vi "select_data_points.vi"(0 "Total HCl masses":dbl[](array[numeric]), 1 "EMFs":dbl[](array[numeric]), 2 "E0":dbl, 3 "k":dbl, 4 "Sample Mass":dbl) -> (5 "EMF Array (pH3-3.5)":dbl[](array[numeric]), 6 "m/m0 Array":dbl[](array[numeric]), 7 "First Point":dbl, 8 "Last Point":dbl)   [LabVIEW 2010]
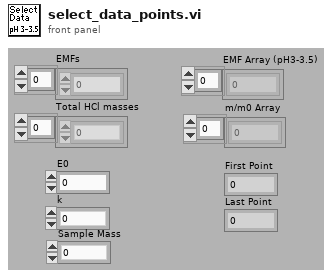
[diagram p1: front panel]
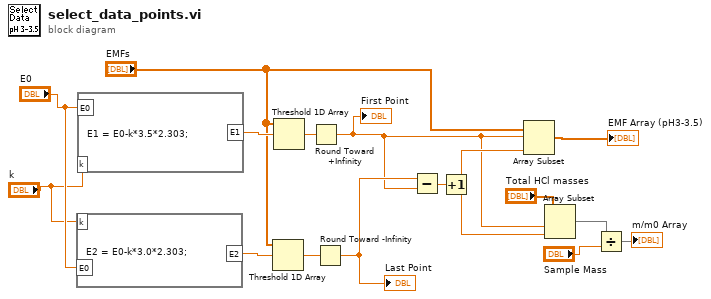
[diagram p0: block diagram]
diagram:
  n1 = formula code="E2 = E0-k*3.0*2.303;"("E0"="E0", "k"="k") -> ("E2"=w12:dbl)
  n2 = formula code="E1 = E0-k*3.5*2.303;"("E0"="E0", "k"="k") -> ("E1"=w13:dbl)
  n3 = Threshold 1D Array(2:w12, 3:"EMFs") -> (0:w10:dbl)  [unwired: 1 in]
  n4 = Threshold 1D Array(2:w13, 3:"EMFs") -> (0:w11:dbl)  [unwired: 1 in]
  n5 = Round Toward +Infinity(x=w11) -> (ceil(x): smallest int >= x=w4:dbl)
  "First Point" <- w4
  n6 = Round Toward -Infinity(1:w10) -> (0:w5:dbl)
  "Last Point" <- w5
  n7 = Subtract(x=w5, y=w4) -> (x-y=w16:dbl)
  n8 = Increment(x=w16) -> (x+1=w15:dbl)
  n9 = Array Subset(array="EMFs", index=w4, length=w15) -> (→"EMF Array (pH3-3.5)":dbl[])
  n10 = Array Subset(array="Total HCl masses", index=w4, length=w15) -> (w14:dbl[])
  n11 = Divide(x=w14, y="Sample Mass") -> (x/y=→"m/m0 Array":dbl[])
